vi "WriteToInstruments.vi"(3 "error in":errorcluster, 4 "New inst. values":cluster{"INST #":string, "Value":dbl}[](array[cluster]), 5 "Inst. array in":cluster{"Inst. #":string, "Value":dbl}[](array[cluster])) -> (0 "error out":errorcluster, 2 "Updated inst. array out":cluster{"Inst. #":string, "Value":dbl}[](array[cluster]))   [LabVIEW 2020]
uses:
  <vilib>/ErrorRing/Error Ring.xnode
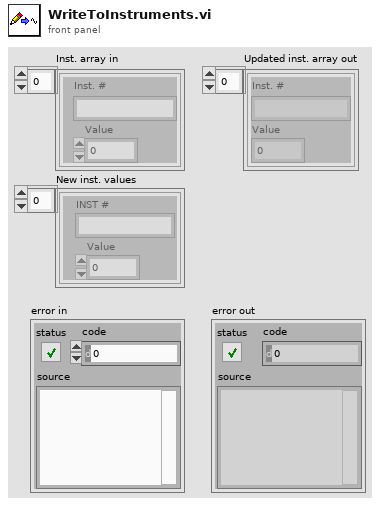
[diagram p1: front panel]
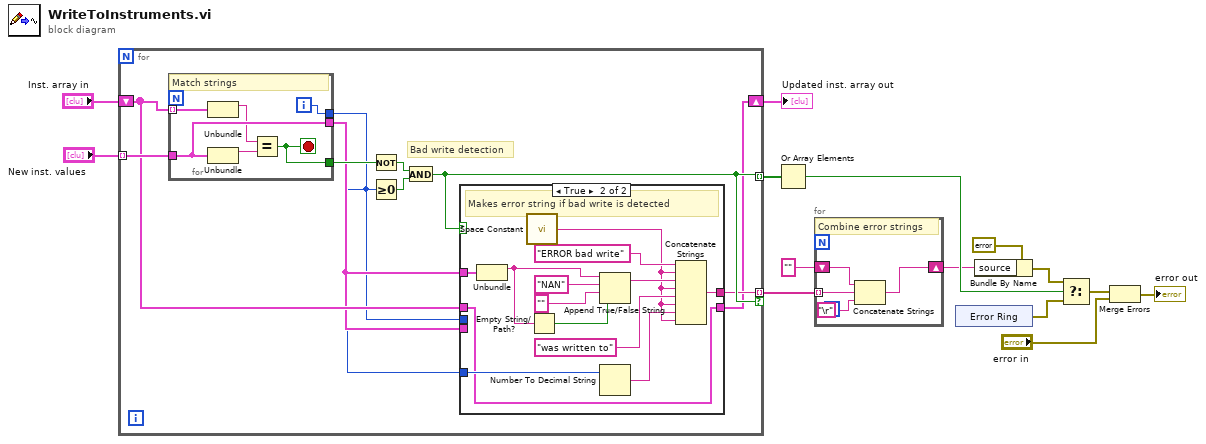
[diagram p0: block diagram]
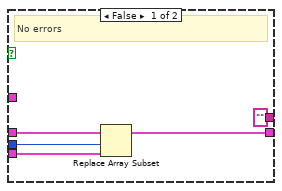
[diagram p2: hidden frame]
diagram:
  n1 = for {
    tunnel: "New inst. values" -> [w24] mode=indexing
    shift-right: [w15] -> w6
    shift-left: "Inst. array in" -> [w18]
    tunnel: [w19] -> w10 mode=indexing if=w20
    tunnel: [w20] -> w13 mode=indexing
    # "Bad write detection"
    n2 = for {
      tunnel: w24 -> [w47]
      tunnel: w18 -> [w48] mode=indexing
      tunnel: [w47] -> w17
      tunnel: [w46] -> w16
      tunnel: [w45] -> w21
      i -> [w46]
      stop <- w45 stop-if-true
      # "Match strings"
      n3 = Unbundle(w48) -> ("Inst. #"=w44:string)  [unwired: 1 out]
      n4 = Unbundle(w47) -> ("INST #"=w43:string)  [unwired: 1 out]
      n5 = Equal?(x=w44, y=w43) -> (x = y?=w45:bool)
    }
    n6 = Not(x=w21) -> (.not. x?=w22:bool)
    n7 = Greater Or Equal To 0?(x=w16) -> (x >= 0?=w23:bool)
    n8 = And(x=w22, y=w23) -> (x .and. y?=w20:bool)
    n9 = case shown="True" w20 {
      tunnel: w17 -> [_ w42]
      tunnel: ["" ("Inst. #") w40] -> w19
      tunnel: w16 -> [_ w33]
      tunnel: w18 -> [w28 w30]
      tunnel: w17 -> [w27 _]
      tunnel: w16 -> [w26 _]
      tunnel: [w25 w30] -> w15
      frame False {
        # "No errors"
        n10 = Replace Array Subset(array=w28, new element=w27, index=w26) -> (w25:cluster{"Inst. #":string, "Value":dbl}[])
      }
      frame True {
        # "Makes error string if bad write is detected"
        n11 = Unbundle(w42) -> ("INST #"=w34:string)  [unwired: 1 out]
        n12 = call <vilib>:"Space Constant.vi"() -> ("String"=w31:string)
        n13 = Empty String/Path?(string/path=w34) -> (empty?=w35:bool)
        n14 = Append True/False String(1:w35, 2:"" ("false string"), 3:"NAN" ("true string"), 4:w34) -> (0:w37:string)
        n15 = Number To Decimal String(number=w33) -> (decimal integer string=w32:string)  [unwired: 1 in]
        n16 = Concatenate Strings("ERROR bad write" ("string"), w31, w37, w31, "was written to" ("string"), w31, w32, w31) -> (w40:string)
      }
    }
  }
  "Updated inst. array out" <- w6
  n17 = Or Array Elements(Boolean array=w13) -> (logical OR=w12:bool)
  n18 = for {
    shift-right: [w50] -> w9
    shift-left: "" -> [w51]
    tunnel: w10 -> [w52] mode=indexing
    # "Combine error strings"
    n19 = Concatenate Strings(w51, w52, "\r") -> (w50:string)
  }
  n20 = xnode "Error Ring"() -> ("error out"=w14:errorcluster)
  n21 = Bundle By Name(cluster=errorcluster {"status"=TRUE, "code"=0, "source"=""} ("error constant"), "source"=w9) -> (w8:errorcluster)
  n22 = Select(t=w8, s=w12, f=w14) -> (s? t:f=w3:errorcluster)
  n23 = Merge Errors(w3, "error in") -> (→"error out":errorcluster)
